vi "Measure.vi"(8 "Error In":errorcluster) -> (0 "Error Out":errorcluster, 2 "RGBU":u16[](array[numeric]), 3 "Luminosity":dbl)   [LabVIEW 2018]
uses:
  <vilib>/myRIO/Instrument Drivers/Onboard IO/I2C/typedefs/I2C User Configuration.ctl
  <vilib>/myRIO/Instrument Drivers/Onboard IO/I2C/typedefs/I2C Transfer Rate.ctl
  <vilib>/myRIO/Instrument Drivers/Onboard IO/I2C/typedefs/I2C Reference.ctl
  <vilib>/myRIO/Common/Instrument Driver Framework/Utilities/typedefs/myRIO Generic Hardware Reference.ctl
  <vilib>/myRIO/Common/Instrument Driver Framework/Utilities/typedefs/Hardware Version Enum.ctl
  <vilib>/myRIO/Common/Instrument Driver Framework/Utilities/typedefs/myRIO v1.0 Reference.ctl
  <vilib>/myRIO/Common/Instrument Driver Framework/Utilities/typedefs/Generic FPGA Reference.ctl
  <vilib>/myRIO/Common/Instrument Driver Framework/myRIO v1.0/I2C/typedefs/I2C Channels Enum.ctl
  <vilib>/myRIO/Instrument Drivers/Onboard IO/I2C/typedefs/I2C Configuration.ctl
  <vilib>/userdefined/High Color/nirio_resource_hc.ctl
  <vilib>/myRIO/Common/Instrument Driver Framework/Utilities/vis/Is FPGA Ref Available.vi
  <vilib>/myRIO/Common/Instrument Driver Framework/myRIO v1.0/I2C/vis/myRIO v1.1 Open I2C.vi
  <vilib>/myRIO/Instrument Drivers/Onboard IO/I2C/vis/Configure.vi
  <vilib>/myRIO/Instrument Drivers/Onboard IO/I2C/vis/Write.vi
  <vilib>/myRIO/Common/Instrument Driver Framework/Utilities/vis/Validate Channels.vi
  <vilib>/myRIO/Common/Instrument Driver Framework/myRIO v1.0/I2C/vis/myRIO v1.0 Reserve I2C.vi
  <vilib>/myRIO/Common/Instrument Driver Framework/myRIO v1.0/I2C/vis/myRIO v1.0 Build MUX Configuration I2C.vi
  <vilib>/myRIO/Common/Instrument Driver Framework/myRIO v1.0/Resource Manager/vis/myRIO v1.0 Reserve Channel List.vi
  <vilib>/myRIO/Common/Instrument Driver Framework/myRIO v1.0/Resource Manager/vis/myRIO v1.0 Create Configuration List.vi
  <vilib>/myRIO/Common/Instrument Driver Framework/myRIO v1.0/Resource Manager/vis/myRIO v1.0 Reserve Channel.vi
  <vilib>/myRIO/Common/Instrument Driver Framework/myRIO v1.0/Resource Manager/vis/myRIO v1.0 Unreserve Channel.vi
  <vilib>/myRIO/Common/Instrument Driver Framework/myRIO v1.0/Resource Manager/vis/myRIO v1.0 Build Mutex Name.vi
  <vilib>/Utility/VariantDataType/GetNumericInfo.vi
  <vilib>/Utility/error.llb/Error Cluster From Error Code.vi
  <vilib>/myRIO/Common/Instrument Driver Framework/myRIO v1.0/myRIO v1.1 Open.vi
  <vilib>/myRIO/Common/Instrument Driver Framework/Utilities/vis/IO Manager.vi
  <vilib>/myRIO/Common/Instrument Driver Framework/Utilities/vis/Configuration Manager.vi
  <vilib>/myRIO/Common/Instrument Driver Framework/myRIO v1.0/Resource Manager/vis/myRIO v1.0 Configure IO.vi
  <vilib>/myRIO/Common/Instrument Driver Framework/myRIO v1.0/myRIO v1.0 Close.vi
  <vilib>/myRIO/Common/Instrument Driver Framework/myRIO v1.0/I2C/vis/myRIO v1.0 Configure I2C.vi
  <vilib>/myRIO/Common/Instrument Driver Framework/myRIO v1.0/I2C/vis/myRIO v1.0 Write I2C.vi
  <vilib>/myRIO/Express VI/Onboard IO/I2C/I2C Express VI.xnode
  <vilib>/myRIO/Instrument Drivers/Onboard IO/I2C/vis/myRIO I2C Open.xnode
  <vilib>/myRIO/Instrument Drivers/Onboard IO/I2C/I2C.lvlib
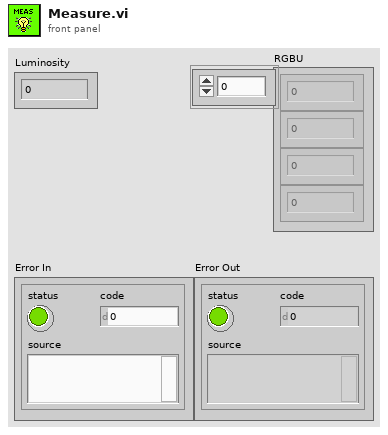
[diagram p1: front panel]
types:
  T1 = enum8{"Clear_L", "Clear_H", "Red_L", "Red_H", "Green_L", "Green_H", "Blue_L", "Blue_H"}[]
  T2 = typedef "I2C.lvlib/I2C Reference.ctl" = cluster{"myRIO Reference":T3, "I2C Channels Enum":T7, "I2C Configuration":T8}
  T3 = typedef "myRIO Generic Hardware Reference.ctl" = cluster{"myRIO Model":T4, "myRIO Hardware Reference":T5}
  T4 = typedef "Hardware Version Enum.ctl" = enum16{"Unknown", "myRIO-1900", "myRIO-1950", "roboRIO", "NI ELVIS RIO CM", "ELVIS III"}
  T5 = typedef "myRIO v1.0 Reference.ctl" = cluster{"Generic FPGA Reference":T6, "Allow multiple opens":bool}
  T6 = typedef "Generic FPGA Reference.ctl" = refnum<k20>
  T7 = typedef "I2C Channels Enum.ctl" = enum16{"Not Connected", "A/I2C", "B/I2C", "I2C/I2C"}
  T8 = typedef "I2C.lvlib/I2C Configuration.ctl" = cluster{"I2C Transfer Rate":T9}
  T9 = typedef "I2C.lvlib/I2C Transfer Rate.ctl" = enum16{"Standard mode (100 kbps)", "Fast mode (400 kbps)"}
  T10 = typedef "I2C.lvlib/I2C User Configuration.ctl" = cluster{"I2C Transfer Rate":T9}
  T11 = typedef "nirio_resource_hc.ctl" = tag
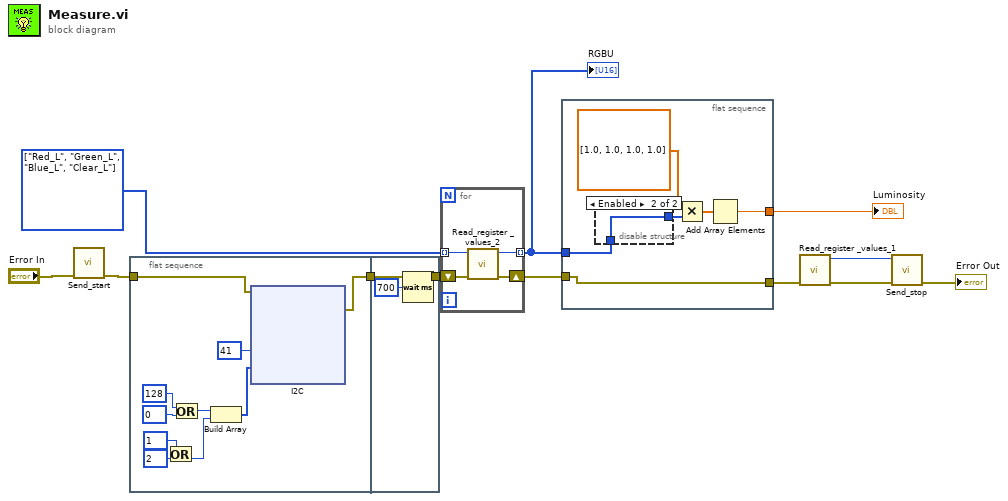
[diagram p0: block diagram]
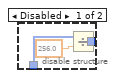
[diagram p2: hidden frame]
diagram:
  w12 = T1 [enum."Red_L", enum."Green_L", enum."Blue_L", enum."Clear_L"] items=["Clear_L", "Clear_H", "Red_L", "Red_H", "Green_L", "Green_H", "Blue_L", "Blue_H"]
  n1 = call "Send_start.vi"("error in"="Error In") -> ("error out"=w8:errorcluster)  [unwired: 10 in]
  n2 = flat-sequence {
    tunnel: w8 -> [w14]
    tunnel: [w13] -> w1
    tunnel: [w62] -> w7
    tunnel: w1 -> [w62]
    frame #0 {
      n3 = Or(x=u8 1 ("Slave Address (7-bit)"), y=u8 2 ("Slave Address (7-bit)")) -> (x .or. y?=w16:u8)
      n4 = Or(x=u8 128 ("Slave Address (7-bit)"), y=u8 0 ("Slave Address (7-bit)")) -> (x .or. y?=w21:u8)
      n5 = Build Array(w21, w16) -> (w17:u8[])
      n6 = xnode "I2C"("Slave Address (7-bit)"=u8 41, "Bytes to Write"=w17, "error in (no error)"=w14) -> ("error out"=w13:errorcluster)
    }
    frame #1 {
      n7 = Wait (ms)(milliseconds to wait=u32 700) -> ()  [unwired: 1 out]
    }
  }
  n8 = for {
    tunnel: w12 -> [w65] mode=indexing
    shift-right: [w64] -> w6
    shift-left: w7 -> [w66]
    tunnel: [w63] -> w10 mode=indexing
    n9 = call "Read_register _values_2.vi"("error in"=w66, "Register"=w65) -> ("error out"=w64:errorcluster, "Data"=w63:u16)  [unwired: 8 in]
  }
  "RGBU" <- w10
  n10 = flat-sequence {
    tunnel: w10 -> [w72]
    tunnel: [w70] -> w9
    tunnel: w6 -> [w67]
    tunnel: [w67] -> w5
    frame #0 {
      n11 = disable-structure shown="Enabled" {
        disable-tunnel: w72 -> [w75 w76]
        disable-tunnel: [w74 w76] -> w68
        frame Disabled {
          n12 = Divide(x=w75, y=256.0) -> (x/y=w74:dbl[])
        }
        frame Enabled {
        }
      }
      n13 = Multiply(x=dbl[] [1.0, 1.0, 1.0, 1.0], y=w68) -> (x*y=w69:dbl[])
      n14 = Add Array Elements(numeric array=w69) -> (sum=w70:dbl)
    }
  }
  n15 = call "Read_register _values_1.vi"("error in"=w5) -> ("error out"=w4:errorcluster, "Data"=w3:u8)  [unwired: 9 in]
  n16 = call "Send_stop.vi"("error in"=w4, "Register value"=w3) -> ("error out"=→"Error Out":errorcluster)  [unwired: 9 in]
  "Luminosity" <- w9
